vi "LoadStaleFiles.vi"(8 "error in (no error)":errorcluster, 10 "config":T1, 11 "Qbus":refnum<class "Qbus.lvclass">) -> (0 "error out":errorcluster)   [LabVIEW 2017, in "FileManager.lvlib"]
uses:
  <vilib>/addons/InsightCM/Devices/Shared/Common/FileManager/FileManager.lvlib
  <vilib>/addons/Qbus/Qbus.lvclass
  <vilib>/addons/InsightCM/Devices/Shared/Common/FileManager/controls/config.ctl
  <vilib>/addons/InsightCM/Utilities/GlobalConfiguration/GlobalConfiguration.lvlib
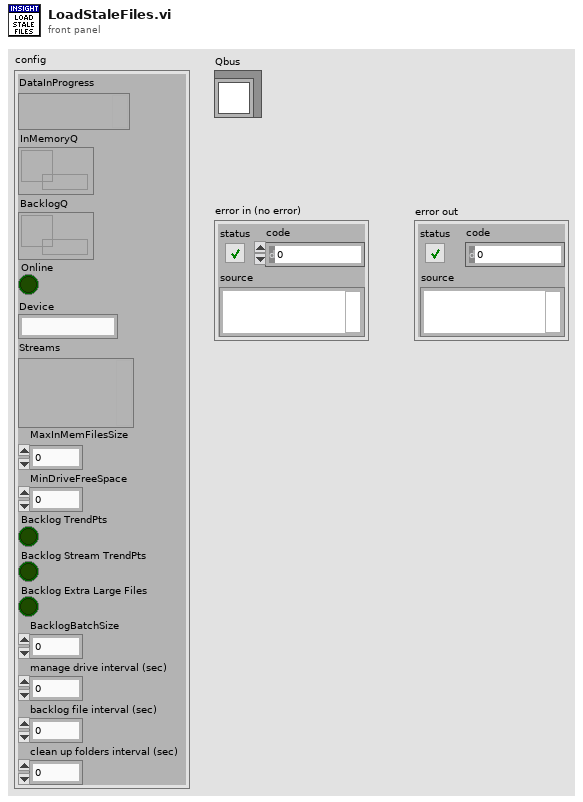
[diagram p1: front panel]
types:
  T1 = typedef "FileManager.lvlib/config.ctl" = cluster{"DataInProgress":variant, "InMemoryQ":refnum<queue>, "BacklogQ":refnum<queue>, "Online":bool, "Device":string, "Streams":variant, "MaxInMemFilesSize":i32, "MinDriveFreeSpace":i32, "Backlog TrendPts":bool, "Backlog Stream TrendPts":bool, "Backlog Extra Large Files":bool, "BacklogBatchSize":i32, "manage drive interval (sec)":dbl, "backlog file interval (sec)":dbl, "clean up folders interval (sec)":dbl}
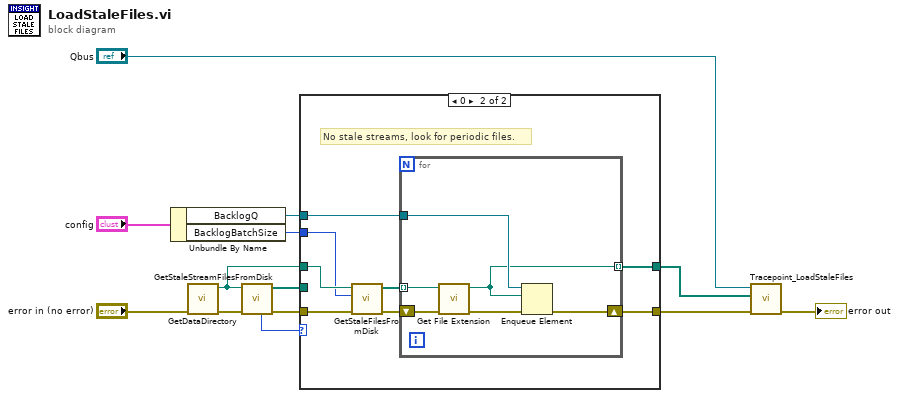
[diagram p0: block diagram]
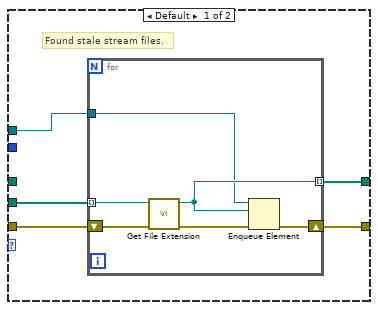
[diagram p2: hidden frame]
diagram:
  n1 = Unbundle By Name("config") -> ("BacklogQ"=w1:refnum<queue>, "BacklogBatchSize"=w3:i32)
  n2 = call <vilib>:"GetDataDirectory.vi"("error in (no error)"="error in (no error)") -> ("error out"=w12:errorcluster, "data directory"=w9:path)  [unwired: 9 in]
  n3 = call <vilib>:"GetStaleStreamFilesFromDisk.vi"("error in (no error)"=w12, "data directory"=w9) -> ("error out"=w13:errorcluster, "file paths"=w8:path[], "files found"=w10:i32)  [unwired: 5 in, 2 out]
  n4 = case shown="0" w10 {
    tunnel: w9 -> [_ w29]
    tunnel: w13 -> [w18 w32]
    tunnel: [w17 w30] -> w7
    tunnel: w8 -> [w16 _]
    tunnel: [w15 w27] -> w4
    tunnel: w3 -> [_ w26]
    tunnel: w1 -> [w14 w25]
    frame Default {
      # "Found stale stream files."
      # "Found stale stream files"
      n5 = for {
        tunnel: w16 -> [w23] mode=indexing
        shift-right: [w24] -> w17
        shift-left: w18 -> [w22]
        tunnel: [w20] -> w15 mode=indexing
        tunnel: w14 -> [w19]
        n6 = call <vilib>:"Get File Extension.vi"("error in (no error)"=w22, "file"=w23) -> ("error out"=w21:errorcluster, "dup file"=w20:path)  [unwired: 5 in, 3 out]
        n7 = Enqueue Element(queue=w19, element=w20, error in (no error)=w21) -> (error out=w24:errorcluster)  [unwired: 1 in, 2 out]
      }
    }
    frame 0 {
      # "No stale streams, look for periodic files."
      # "No Stream Files. Load periodic ones"
      n8 = call <vilib>:"GetStaleFilesFromDisk.vi"("error in (no error)"=w32, "BacklogBatchSize"=w26, "data directory"=w29) -> ("error out"=w31:errorcluster, "file paths"=w28:path[])  [unwired: 6 in, 1 out]
      n9 = for {
        tunnel: w28 -> [w36] mode=indexing
        shift-right: [w38] -> w30
        shift-left: w31 -> [w35]
        tunnel: w25 -> [w37]
        tunnel: [w33] -> w27 mode=indexing
        n10 = call <vilib>:"Get File Extension.vi"("error in (no error)"=w35, "file"=w36) -> ("error out"=w34:errorcluster, "dup file"=w33:path)  [unwired: 5 in, 3 out]
        n11 = Enqueue Element(queue=w37, element=w33, error in (no error)=w34) -> (error out=w38:errorcluster)  [unwired: 1 in, 2 out]
      }
    }
  }
  n12 = call <vilib>:"Tracepoint_LoadStaleFiles.vi"("error in (no error)"=w7, "file paths"=w4, "Qbus in"="Qbus") -> ("error out"=→"error out":errorcluster)  [unwired: 8 in]
